vi "Cross-Talk, Calculate Differential with Waveform 4.vi"(0 "Waveform Array In":waveform(dbl)[](array[waveform]), 7 "Idle Offset Voltage":dbl) -> (4 "Waveform Array Out":waveform(dbl)[](array[waveform]))   [LabVIEW 2010]
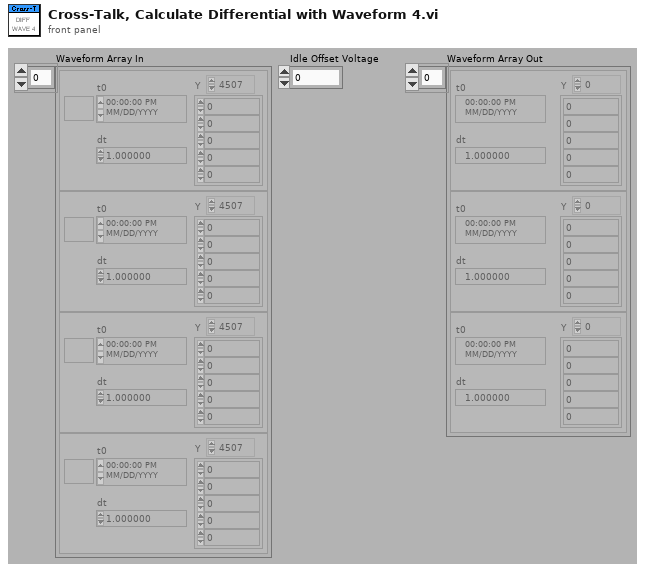
[diagram p1: front panel]
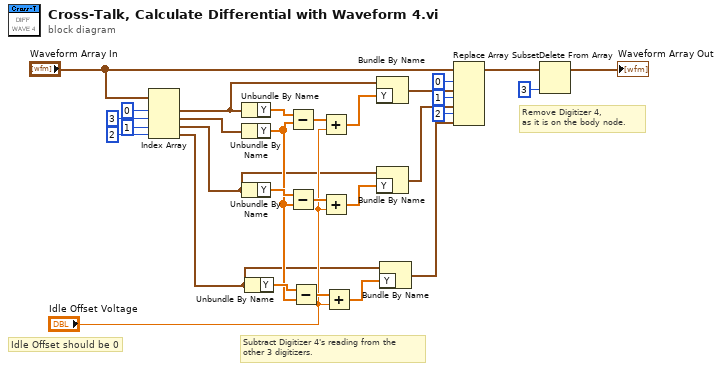
[diagram p0: block diagram]
diagram:
  # "Subtract Digitizer 4's reading from the\nother 3 digitizers."
  # "Idle Offset should be 0"
  # "Remove Digitizer 4,\nas it is on the body node."
  n1 = Index Array(array="Waveform Array In", index #1=0 ("index"), index #2=3 ("index"), index #3=1 ("index"), index #4=2 ("index")) -> (element #1=w24:waveform(dbl), element #2=w14:waveform(dbl), element #3=w9:waveform(dbl), element #4=w8:waveform(dbl))
  n2 = Unbundle By Name(w24) -> ("Y"=w27:dbl[])
  n3 = Unbundle By Name(w14) -> ("Y"=w13:dbl[])
  n4 = Unbundle By Name(w9) -> ("Y"=w20:dbl[])
  n5 = Unbundle By Name(w8) -> ("Y"=w17:dbl[])
  n6 = Subtract(x=w27, y=w13) -> (x-y=w26:dbl[])
  n7 = Subtract(x=w20, y=w13) -> (x-y=w19:dbl[])
  n8 = Subtract(x=w17, y=w13) -> (x-y=w16:dbl[])
  n9 = Add(x=w26, y="Idle Offset Voltage") -> (x+y=w25:dbl[])
  n10 = Add(x=w19, y="Idle Offset Voltage") -> (x+y=w18:dbl[])
  n11 = Add(x=w16, y="Idle Offset Voltage") -> (x+y=w15:dbl[])
  n12 = Bundle By Name(cluster=w24, "Y"=w25) -> (w22:waveform(dbl))
  n13 = Bundle By Name(cluster=w9, "Y"=w18) -> (w7:waveform(dbl))
  n14 = Bundle By Name(cluster=w8, "Y"=w15) -> (w6:waveform(dbl))
  n15 = Replace Array Subset(array="Waveform Array In", new element #1=w22, index #1=0 ("index"), new element #2=w7, index #2=1 ("index"), new element #3=w6, index #3=2 ("index")) -> (w3:waveform(dbl)[])
  n16 = Delete From Array(array=w3, index=3) -> (array with subset deleted=→"Waveform Array Out":waveform(dbl)[])  [unwired: 1 in, 1 out]
